vi "T1 Parametric Testing Retrieval.vi"(8 "error in (no error)":errorcluster, 10 "table name":string="Test_Results", 11 "connection reference":T1) -> (0 "error out":errorcluster, 3 "connection reference out":T1)   [LabVIEW 2018]
doc: "The T1 Parametric testing application performs parametric testing of T1 signals. The T1 signal is a 1.544 Mb/s pulsed digital signal formed by multiplexing 24 voice channels. Each channel is sampled at 8000 samples/sec. Each sample is then converted to 8 bits using Pulse Coded Multiplexing. The 24 channels are then time-division multiplexed. Each frame, which corresponds to one sampling period, contains 192 bits ( 8 times 24) plus one bit for frame synchronization. Since frames occur at 8000 times per second, the bit rate is 1.544 Mb/s\n\nThis application performs the following parametric tests on T1 signals:\n\n1. Mask Test: Compares T1 signals with standard masks. The type of masks that are supported are ITU G.703 mask, EIA/TIA 547 and ANSI T1.102. The graph shows the mask in grey, the actual signal in green and failures as red squares. A boolean indicates whether the signal passed or failed the mask test and the indicator Number of Hits shows the number of times the signal did not pass the mask test.\n\n2. Measure T1 signal amplitude : Measures the amplitude of the T1 signal. The peak amplitude is displayed in the indicator Measured Amplitude.\n\n3. Measure T1 signal frequency : Measures the frequency of the T1 signal. The signal frequency in MHz is displayed in the indicator Measured Frequency."
uses:
  <vilib>/addons/database/Connection.llb/Conn ObjectReference.ctl
  <vilib>/addons/database/Connection.llb/Conn Execute.vi
  <vilib>/addons/database/Recordset.llb/Rec Fetch Recordset Data (R).vi
  <vilib>/addons/database/Recordset.llb/Rec Destroy - Connection.vi
  <vilib>/addons/database/Recordset.llb/Rec Save Recordset To File (R).vi
  <vilib>/addons/database/_DB Variant To Data/Database Variant To Data.xnode
  <vilib>/addons/database/NI_Database_API.lvlib
panel:
  in  "Sort By":u16(ring) items=["Operator", "Date/Time", "UUT Serial #", "Pass/Fail"]
  in  "File Name":path=path "c:/test data.xml"
  in  "Order":u16(ring) items=["Ascending", "Descending"]
  out "Database Data":i32(listbox)=-1
  in  "quit":bool
  in  "Retrieve Only Failures":bool
  in  "Retrieve All Data":bool
  in  "Sort Data":bool
  in  "Export All Data to XML":bool
  # "Telecommunications Parametric Testing Data Retrieval"
  # "Instructions: Click Get Data, then try the various other operations on the data. Click Quit when done."
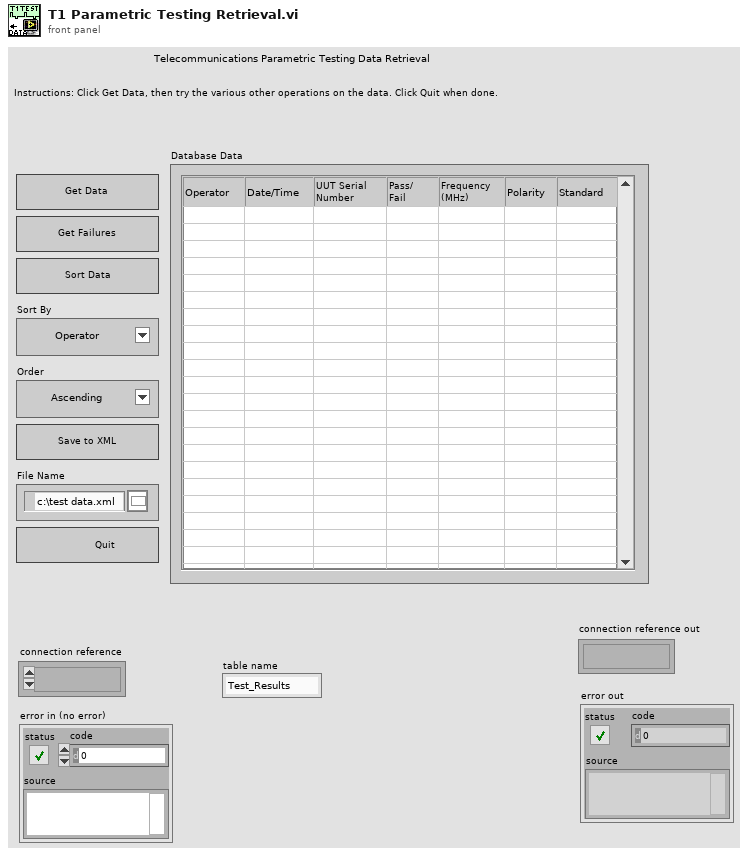
[diagram p1: front panel]
types:
  T1 = typedef "NI_Database_API.lvlib/Conn ObjectReference.ctl" = refnum<k1>
  T2 = typedef "NI_Database_API.lvlib/Rec ObjectReference.ctl" = refnum<k1>
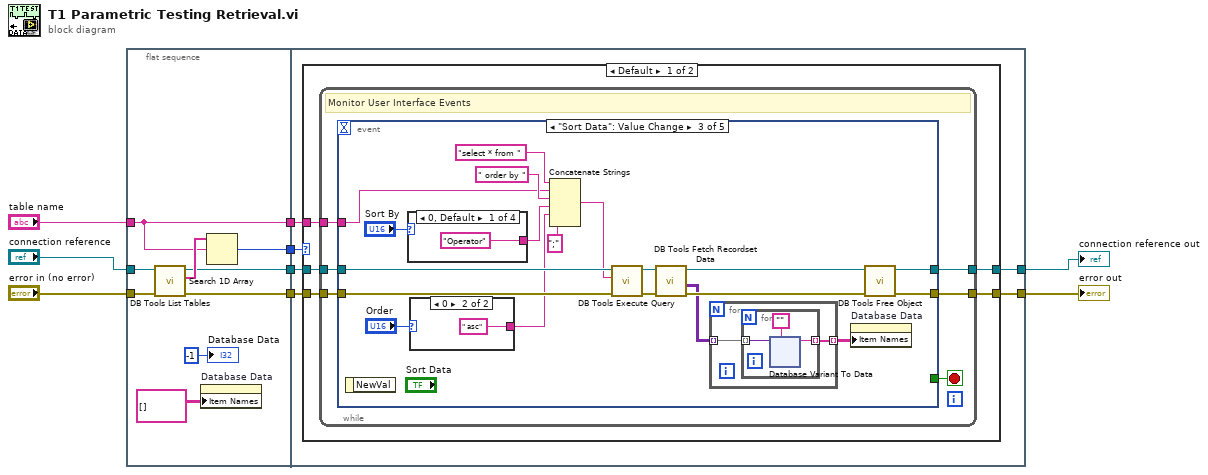
[diagram p0: block diagram]
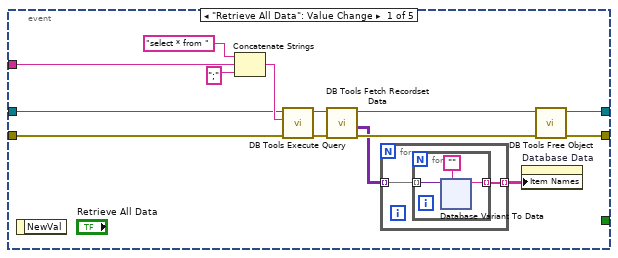
[diagram p2: hidden frame]
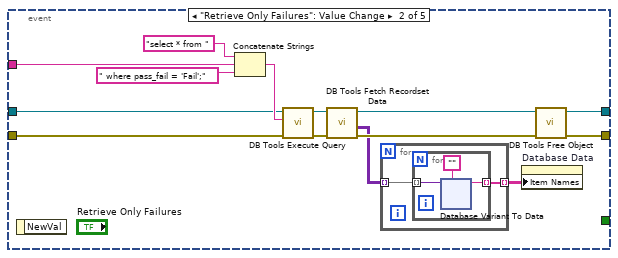
[diagram p3: hidden frame]
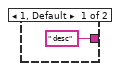
[diagram p4: hidden frame]
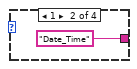
[diagram p5: hidden frame]
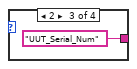
[diagram p6: hidden frame]
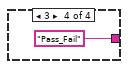
[diagram p7: hidden frame]
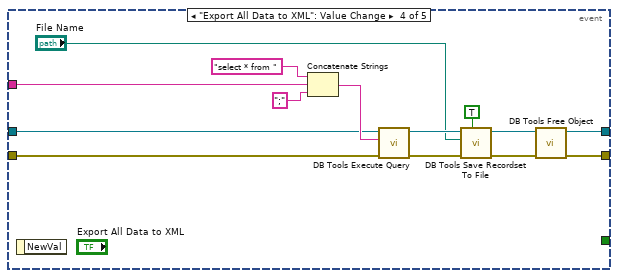
[diagram p8: hidden frame]
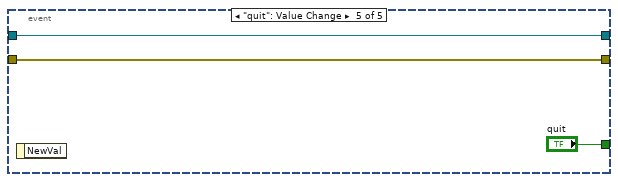
[diagram p9: hidden frame]
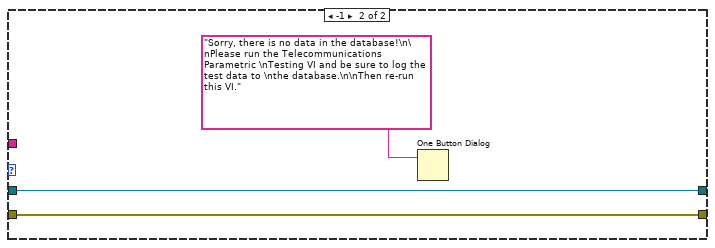
[diagram p10: hidden frame]
diagram:
  n1 = flat-sequence {
    tunnel: [w15] -> w9
    tunnel: "table name" -> [w10]
    tunnel: "connection reference" -> [w14]
    tunnel: "error in (no error)" -> [w13]
    tunnel: [w12] -> w5
    tunnel: [w11] -> w4
    tunnel: [w10] -> w1
    tunnel: w9 -> [w24]
    tunnel: w5 -> [w23]
    tunnel: w4 -> [w22]
    tunnel: [w21] -> w2
    tunnel: [w20] -> w3
    tunnel: w1 -> [w19]
    frame #0 {
      n2 = call <vilib>:"DB Tools List Tables.vi"("error in (no error)"=w13, "connection reference"=w14) -> ("error out"=w12:errorcluster, "tables"=w16:string[], "connection reference out"=w11:T1)  [unwired: 3 in]
      n3 = property on="Database Data" class="MCListbox (strict)"("Item Names"=string[][] []) -> ()  [unwired: 2 in, 2 out]
      n4 = Search 1D Array(1D array=w16, element=w10) -> (index of element=w15:i32)  [unwired: 1 in]
      "Database Data" <- -1 ("Database Data")
    }
    frame #1 {
      n5 = case shown="Default" w24 {
        tunnel: w23 -> [w29 w218]
        tunnel: w22 -> [w28 w219]
        tunnel: [w27 w219] -> w21
        tunnel: [w26 w218] -> w20
        tunnel: w19 -> [w25 _]
        frame Default {
          n6 = while {
            tunnel: w29 -> [w34]
            tunnel: w28 -> [w35]
            tunnel: [w32] -> w27
            tunnel: [w31] -> w26
            tunnel: w25 -> [w30]
            stop <- w33 stop-if-true
            # "Monitor User Interface Events"
            n7 = event shown="[2] \"Sort Data\": Value Change" {
              selector: _ -> [_ _ _ _ _]
              dyn-events: _ -> [_ _ _ _ _]
              timeout: _ -> [_ _ _ _ _]
              tunnel: w35 -> [w41 w92 w150 w205 w216]
              tunnel: w34 -> [w40 w91 w149 w204 w215]
              tunnel: [_ _ _ _ "quit"] -> w33
              tunnel: [w38 w89 w147 w202 w216] -> w32
              tunnel: [w39 w90 w148 w203 w215] -> w31
              tunnel: w30 -> [w37 w88 w140 w201 _]
              event "Retrieve All Data": Value Change {
                n8 = event-data() -> ()  [unwired: 1 in, 1 out]
                n9 = Concatenate Strings("select * from " ("SQL query"), w37, ";" ("Substring")) -> (w42:string)
                n10 = call-poly <vilib>:"DB Tools Execute Query.vi"("error in (no error)"=w40, "SQL query"=w42, "connection reference"=w41) -> ("error out"=w45:errorcluster, "recordset reference"=w44:T2)  [unwired: 5 in]
                n11 = call-poly <vilib>:"DB Tools Fetch Recordset Data.vi"("error in (no error)"=w45, "recordset reference"=w44) -> ("error out"=w49:errorcluster, "recordset data"=w46:variant[][], "recordset reference out"=w48:T2)  [unwired: 3 in]
                n12 = for {
                  tunnel: w46 -> [w51] mode=indexing
                  tunnel: [w50] -> w47 mode=indexing
                  n13 = for {
                    tunnel: w51 -> [w54] mode=indexing
                    tunnel: [w53] -> w50 mode=indexing
                    n14 = xnode "Database Variant To Data"("database variant"=w54, "type"="") -> ("data"=w53:string)  [unwired: 1 in, 1 out]
                  }
                }
                n15 = property on="Database Data" class="MCListbox (strict)"("Item Names"=w47) -> ()  [unwired: 2 in, 2 out]
                n16 = call-poly <vilib>:"DB Tools Free Object.vi"("error in (no error)"=w49, "recordset reference"=w48) -> ("error out"=w39:errorcluster, "connection reference"=w38:T1)  [unwired: 8 in]
              }
              event "Retrieve Only Failures": Value Change {
                n17 = event-data() -> ()  [unwired: 1 in, 1 out]
                n18 = Concatenate Strings("select * from " ("SQL query"), w88, " where pass_fail = 'Fail';" ("Substring")) -> (w93:string)
                n19 = call-poly <vilib>:"DB Tools Execute Query.vi"("error in (no error)"=w91, "SQL query"=w93, "connection reference"=w92) -> ("error out"=w96:errorcluster, "recordset reference"=w95:T2)  [unwired: 5 in]
                n20 = call-poly <vilib>:"DB Tools Fetch Recordset Data.vi"("error in (no error)"=w96, "recordset reference"=w95) -> ("error out"=w100:errorcluster, "recordset data"=w97:variant[][], "recordset reference out"=w99:T2)  [unwired: 3 in]
                n21 = for {
                  tunnel: w97 -> [w102] mode=indexing
                  tunnel: [w101] -> w98 mode=indexing
                  n22 = for {
                    tunnel: w102 -> [w105] mode=indexing
                    tunnel: [w104] -> w101 mode=indexing
                    n23 = xnode "Database Variant To Data"("database variant"=w105, "type"="") -> ("data"=w104:string)  [unwired: 1 in, 1 out]
                  }
                }
                n24 = property on="Database Data" class="MCListbox (strict)"("Item Names"=w98) -> ()  [unwired: 2 in, 2 out]
                n25 = call-poly <vilib>:"DB Tools Free Object.vi"("error in (no error)"=w100, "recordset reference"=w99) -> ("error out"=w90:errorcluster, "connection reference"=w89:T1)  [unwired: 8 in]
              }
              event "Sort Data": Value Change {
                n26 = event-data() -> ()  [unwired: 1 in, 1 out]
                n27 = case shown="0, Default" "Sort By" {
                  tunnel: ["Operator" ("Substring") "Date_Time" ("Substring") "UUT_Serial_Num" ("Substring") "Pass_Fail" ("Substring")] -> w143
                  frame 0, Default {
                  }
                  frame 1 {
                  }
                  frame 2 {
                  }
                  frame 3 {
                  }
                }
                n28 = case shown="0" "Order" {
                  tunnel: [" desc" ("Substring") " asc" ("Substring")] -> w138
                  frame 1, Default {
                  }
                  frame 0 {
                  }
                }
                n29 = Concatenate Strings("select * from " ("SQL query"), w140, " order by " ("Substring"), w143, w138, ";" ("Substring")) -> (w141:string)
                n30 = call-poly <vilib>:"DB Tools Execute Query.vi"("error in (no error)"=w149, "SQL query"=w141, "connection reference"=w150) -> ("error out"=w152:errorcluster, "recordset reference"=w151:T2)  [unwired: 5 in]
                n31 = call-poly <vilib>:"DB Tools Fetch Recordset Data.vi"("error in (no error)"=w152, "recordset reference"=w151) -> ("error out"=w156:errorcluster, "recordset data"=w153:variant[][], "recordset reference out"=w155:T2)  [unwired: 3 in]
                n32 = for {
                  tunnel: w153 -> [w164] mode=indexing
                  tunnel: [w163] -> w154 mode=indexing
                  n33 = for {
                    tunnel: w164 -> [w167] mode=indexing
                    tunnel: [w166] -> w163 mode=indexing
                    n34 = xnode "Database Variant To Data"("database variant"=w167, "type"="") -> ("data"=w166:string)  [unwired: 1 in, 1 out]
                  }
                }
                n35 = property on="Database Data" class="MCListbox (strict)"("Item Names"=w154) -> ()  [unwired: 2 in, 2 out]
                n36 = call-poly <vilib>:"DB Tools Free Object.vi"("error in (no error)"=w156, "recordset reference"=w155) -> ("error out"=w148:errorcluster, "connection reference"=w147:T1)  [unwired: 8 in]
              }
              event "Export All Data to XML": Value Change {
                n37 = event-data() -> ()  [unwired: 1 in, 1 out]
                n38 = Concatenate Strings("select * from " ("SQL query"), w201, ";" ("Substring")) -> (w211:string)
                n39 = call-poly <vilib>:"DB Tools Execute Query.vi"("error in (no error)"=w204, "SQL query"=w211, "connection reference"=w205) -> ("error out"=w208:errorcluster, "recordset reference"=w207:T2)  [unwired: 5 in]
                n40 = call-poly <vilib>:"DB Tools Save Recordset To File.vi"("overwrite? (F)"=TRUE ("overwrite? (f)"), "error in (no error)"=w208, "file name"="File Name", "recordset reference"=w207) -> ("error out"=w213:errorcluster, "recordset reference out"=w212:T2)  [unwired: 4 in]
                n41 = call-poly <vilib>:"DB Tools Free Object.vi"("error in (no error)"=w213, "recordset reference"=w212) -> ("error out"=w203:errorcluster, "connection reference"=w202:T1)  [unwired: 8 in]
              }
              event "quit": Value Change {
                n42 = event-data() -> ()  [unwired: 1 in, 1 out]
              }
            }
          }
        }
        frame -1 {
          n43 = One Button Dialog(message="Sorry, there is no data in the database!\n\nPlease run the Telecommunications Parametric \nTesting VI and be sure to log the test data to \nthe database.\n\nThen re-run this VI.") -> ()  [unwired: 1 in, 1 out]
        }
      }
    }
  }
  "connection reference out" <- w2
  "error out" <- w3
